vi "Global Stop TempSensor.vi"() -> ()   [LabVIEW 2014]
panel:
  out "Global Stop TempSensor":bool
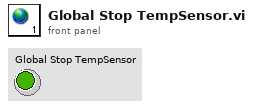
[diagram p1: front panel]
diagram:
